vi "QR_top_left.vi"(8 "errin":errorcluster, 11 "image":string) -> (0 "error out":errorcluster caption="errout", 3 "Réponse":string, 5 "version":string, 6 "SN":string, 7 "PN":string)   [LabVIEW 2020]
uses:
  <userlib>/Alex.vi/FGV.ctl
  <vilib>/regexp/Match Regular Expression.xnode
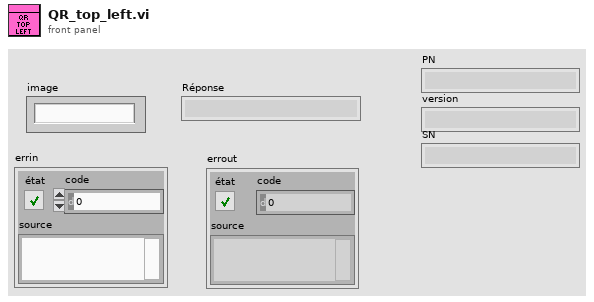
[diagram p1: front panel]
types:
  T1 = typedef "FGV.ctl" = enum16{"GET", "SET", "RAZ"}
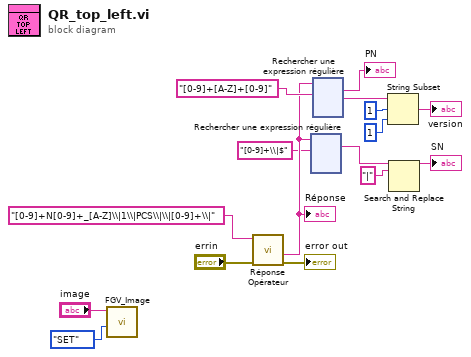
[diagram p0: block diagram]
diagram:
  n1 = call <userlib>:"FGV_Image.vi"("Énum"=FGV."SET", "IN"="image") -> ()  [unwired: 9 in, 1 out]
  n2 = call "Réponse Opérateur.vi"("errin"="errin", "expression régulière"="[0-9]+N[0-9]+_[A-Z]\\|1\\|PCS\\|\\|[0-9]+\\|") -> ("errout"=→"error out":errorcluster, "toute l'expression"=w5:string)  [unwired: 7 in, 1 out]
  "Réponse" <- w5
  n3 = xnode "Rechercher une expression régulière"("chaîne en entrée"=w5, "expression régulière"="[0-9]+\\|$" ("chaîne en entrée")) -> ("toute l'expression"=w3:string)  [unwired: 4 in, 4 out]
  n4 = xnode "Rechercher une expression régulière"("chaîne en entrée"=w5, "expression régulière"="[0-9]+[A-Z]+[0-9]" ("chaîne en entrée")) -> ("toute l'expression"=→"PN":string, "après la correspondance"=w9:string)  [unwired: 4 in, 3 out]
  n5 = String Subset(string=w9, offset (0)=1, length (rest)=1 ("longueur (reste)")) -> (substring=→"version":string)
  n6 = Search and Replace String(input string=w3, search string="|" ("chaîne recherchée")) -> (result string=→"SN":string)  [unwired: 6 in, 3 out]
